vi "Write Actuator.vi"(10 "IActuator.lvclass":refnum<class "IActuator.lvclass">, 11 "Model in":refnum<class "Model.lvclass">) -> (3 "Model out":refnum<class "Model.lvclass">)   [LabVIEW 2015, in "Model.lvclass"]
uses:
  Model.lvclass
  Actuator/IActuator/IActuator.lvclass
  Model.lvclass/Model.ctl
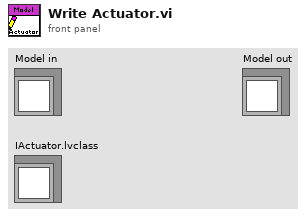
[diagram p1: front panel]
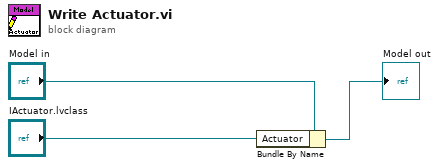
[diagram p0: block diagram]
diagram:
  n1 = Bundle By Name(cluster="Model in", "Actuator"="IActuator.lvclass") -> (→"Model out":refnum<class "Model.lvclass">)
